vi "Update.vi"(8 "error in (no error)":errorcluster, 10 "Message in":refnum<class "UpdateMessage.lvclass">, 11 "DAQMH121119OrcaFlash in":refnum<class "DAQOrcaFlash.lvclass">) -> (0 "error out":errorcluster, 3 "DAQMH121119OrcaFlash out":refnum<class "DAQOrcaFlash.lvclass">)   [LabVIEW 2012, in "DAQOrcaFlash.lvclass"]
doc: "The update method processes the command 'update'. \n\nThe command 'update' is used for receiving new values to be set to the private data of the class. This could be seen as a public set method for setting new parameters to the private class data."
uses:
  DAQOrcaFlash.lvclass
  <vilib>/Distrio/Murmex/UpdateMessage/UpdateMessage.lvclass
  <vilib>/Distrio/Murmex/Murmex/Murmex.lvclass
  visualisation_line_cluster.ctl
  merit_factor_type.ctl
panel:
  # "This method is called when the UPDATE\ntrigger is sent. \n\nOverride this method when your component needs to\nrespond to this trigger. \n\nCall parent for proper implementation"
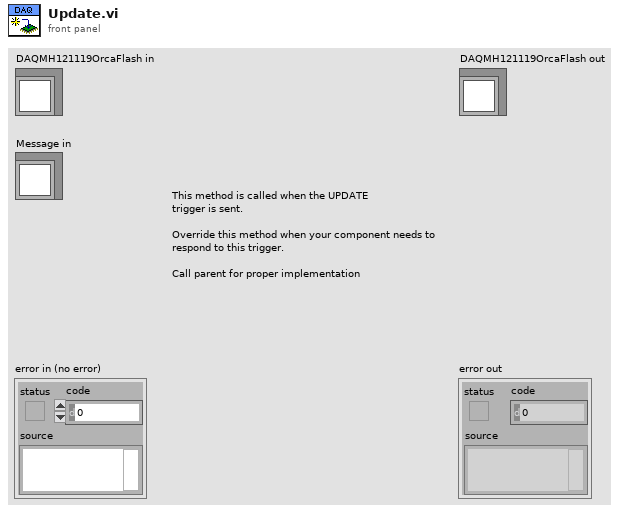
[diagram p1: front panel]
types:
  T1 = typedef "DAQOrcaFlash.lvclass/merit_factor_type.ctl" = enum16{"full frame intensity", "ROI beads", "Weber contrast", "Michelson contrast", "RMS contrast", "Line profile analysis", "ROI analysis", "FFT", "SNR", "5% brightest"}
  T2 = typedef "DAQOrcaFlash.lvclass/visualisation_line_cluster.ctl" = cluster{"direction":enum16{"horizontal", "vertical"}, "position":i32}
  T3 = typedef "IMAQ Image.ctl" = refnum<image>
  T4 = cluster{"Conversion Method":u32, "Minimum Value":i32, "Maximum Value":i32, "# Shifts":i32}
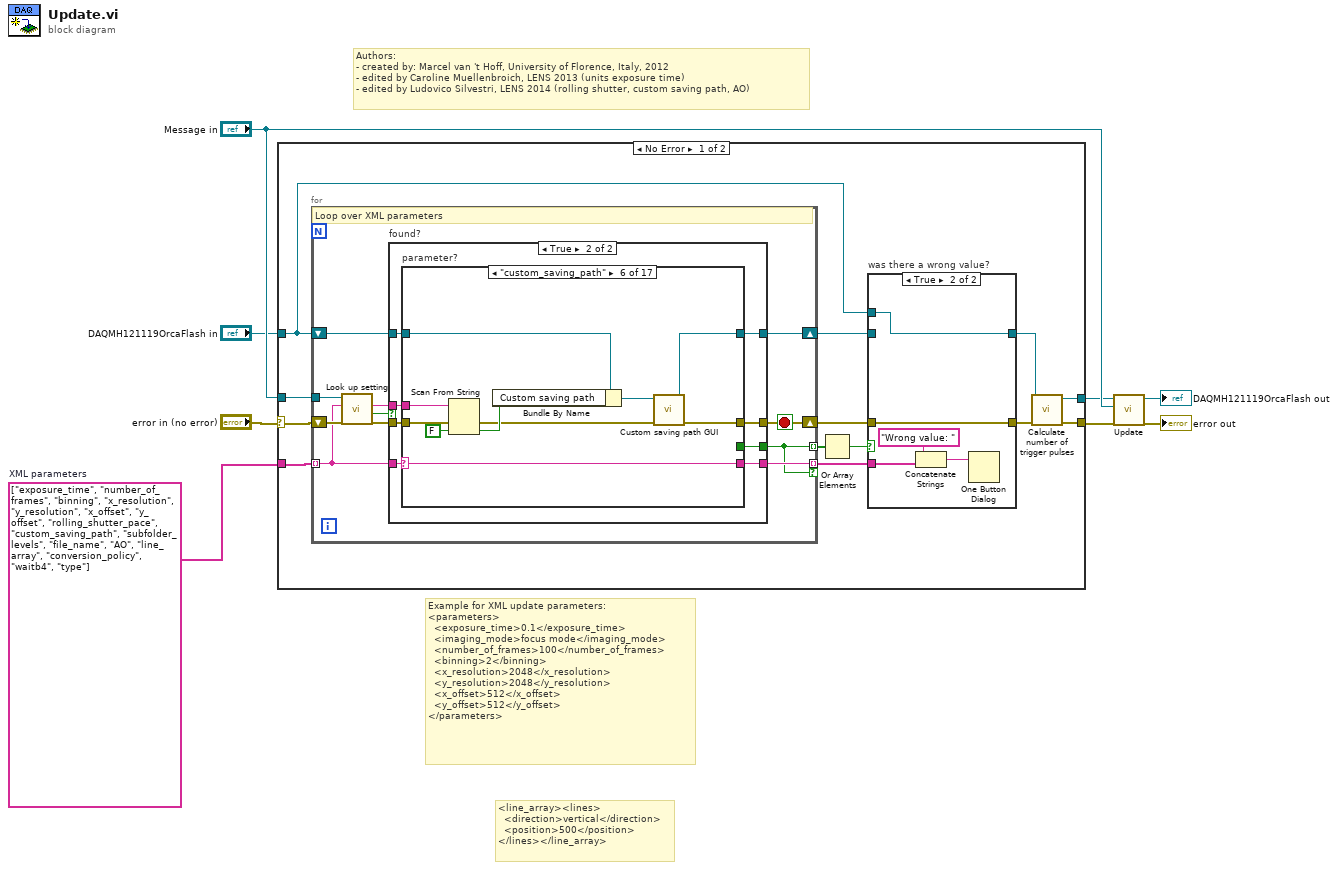
[diagram p0: block diagram]
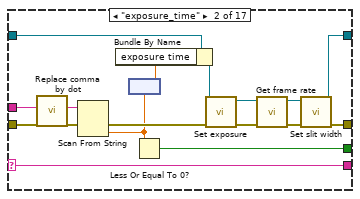
[diagram p5: hidden frame]
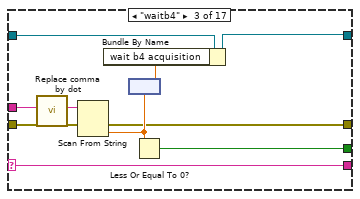
[diagram p6: hidden frame]
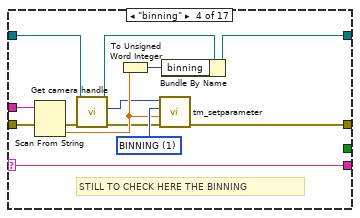
[diagram p7: hidden frame]
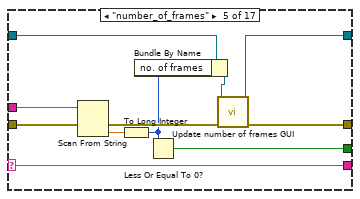
[diagram p8: hidden frame]
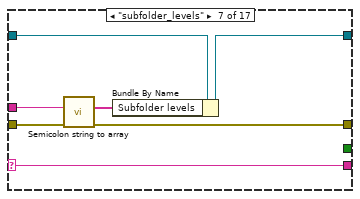
[diagram p9: hidden frame]
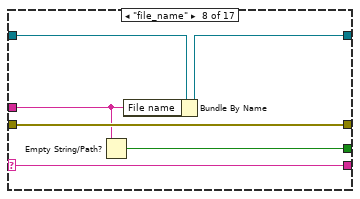
[diagram p10: hidden frame]
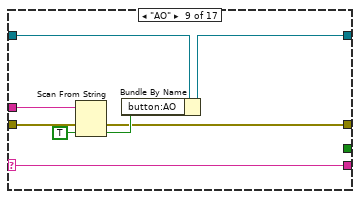
[diagram p11: hidden frame]
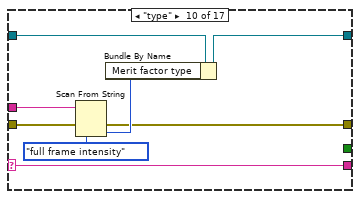
[diagram p12: hidden frame]
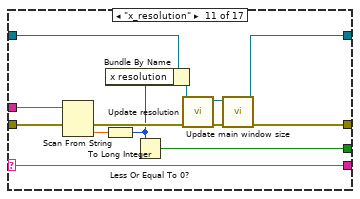
[diagram p13: hidden frame]
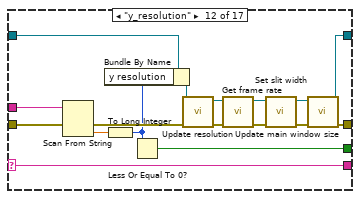
[diagram p14: hidden frame]
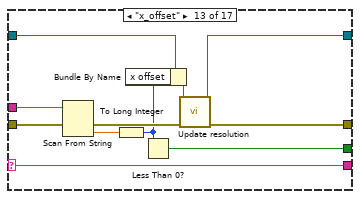
[diagram p15: hidden frame]
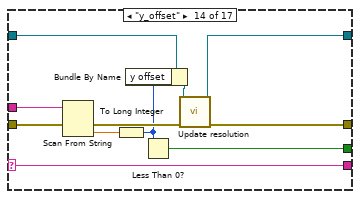
[diagram p16: hidden frame]
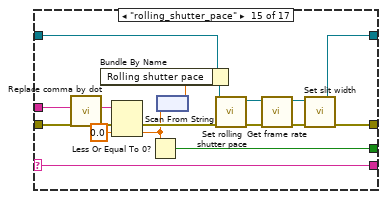
[diagram p17: hidden frame]
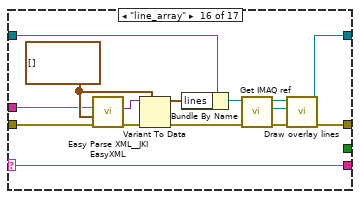
[diagram p18: hidden frame]
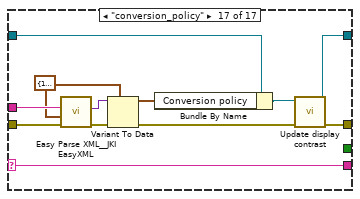
[diagram p19: hidden frame]
diagram:
  w8 = string[] ["exposure_time", "number_of_frames", "binning", "x_resolution", "y_resolution", "x_offset", "y_offset", "rolling_shutter_pace", "custom_saving_path", "subfolder_levels", "file_name", "AO", "line_array", "conversion_policy", "waitb4", "type"]  # XML parameters
  # "<line_array><lines>\n  <direction>vertical</direction>\n  <position>500</position>\n</lines></line_array>"
  # "Example for XML update parameters:\n<parameters>\n  <exposure_time>0.1</exposure_time>\n  <imaging_mode>focus mode</imaging_mode>\n  <number_of_frames>100</number_of_frames>\n  <binning>2</binning>\n  <x_resolution>2048</x_resolution>\n  <y_resolution>2048</y_resolution>\n  <x_offset>512</x_offset>\n  <y_offset>512</y_offset>\n</parameters>"
  # "Authors: \n- created by: Marcel van 't Hoff, University of Florence, Italy, 2012\n- edited by Caroline Muellenbroich, LENS 2013 (units exposure time)\n- edited by Ludovico Silvestri, LENS 2014 (rolling shutter, custom saving path, AO)"
  n1 = case shown="No Error" "error in (no error)" {
    selector: "error in (no error)" -> [w21 w240]
    tunnel: [w18 w240] -> w3
    tunnel: [w17 w239] -> w4
    tunnel: "DAQMH121119OrcaFlash in" -> [w14 w239]
    tunnel: "Message in" -> [w20 _]
    tunnel: w8 -> [w19 _]
    frame No Error {
      n2 = for "loop over parameters" {
        shift-right: [w37] -> w9
        shift-left: w21 -> [w35]
        shift-right: [w38] -> w12
        shift-left: w14 -> [w39]
        tunnel: w20 -> [w36]
        tunnel: w19 -> [w33] mode=indexing
        tunnel: [w29] -> w16 mode=indexing
        tunnel: [w30] -> w11 mode=indexing if=w29
        stop <- w37 stop-if-true
        # "Loop over XML parameters"
        n3 = call <vilib>:"Look up setting.vi"("error in (no error)"=w35, "tag name"=w33, "UpdateMessage in"=w36) -> ("error out"=w34:errorcluster, "found?"=w32:bool, "value"=w31:string)  [unwired: 5 in, 1 out]
        n4 = case "found?" shown="True" w32 {
          tunnel: w34 -> [w41 w50]
          tunnel: w31 -> [_ w49]
          tunnel: w33 -> [w40 w48]
          tunnel: w39 -> [w42 w47]
          tunnel: [w41 w46] -> w37
          tunnel: [w42 w45] -> w38
          tunnel: [_ w44] -> w29
          tunnel: [w40 w43] -> w30
          frame False {
          }
          frame True {
            # "XML parameter found?"
            n5 = case "parameter?" shown="\"custom_saving_path\"" w48 {
              selector: w48 -> [w51 w54 w72 w80 w95 w104 w114 w123 w127 w136 w143 w156 w173 w184 w195 w212 w227]
              tunnel: w50 -> [w52 w69 w79 w92 w102 w110 w118 w124 w133 w142 w153 w170 w181 w192 w210 w222 w235]
              tunnel: w49 -> [_ w68 w78 w91 w101 w111 w116 w122 w132 w141 w154 w171 w182 w193 w200 w223 w236]
              tunnel: w47 -> [w53 w59 w75 w84 w103 w113 w120 w126 w131 w140 w155 w172 w183 w194 w211 w221 w234]
              tunnel: [w52 w63 w71 w86 w98 w107 w117 w124 w128 w137 w149 w159 w177 w189 w205 w214 w231] -> w46
              tunnel: [w53 w62 w70 w90 w96 w105 w119 w125 w129 w138 w147 w161 w176 w187 w204 w216 w230] -> w45
              tunnel: [_ w55 w73 _ w93 _ _ w121 _ _ w144 w157 w174 w185 w196 _ _] -> w44
              tunnel: [w51 w54 w72 w80 w95 w104 w114 w123 w127 w136 w143 w156 w173 w184 w195 w212 w227] -> w43
              frame Default {
              }
              frame "exposure_time" {
                n6 = call <vilib>:"Replace comma by dot.vi"("input string"=w68) -> ("result string"=w66:string)  [unwired: 10 in]
                n7 = Scan From String(input string=w66, error in=w69) -> (error out=w57:errorcluster, output 1=w56:dbl)  [unwired: 3 in, 2 out]
                n8 = node(w56) -> (w67:dbl[unit])
                n9 = Bundle By Name(cluster=w59, "exposure time"=w67) -> (w58:refnum<class "DAQOrcaFlash.lvclass">)
                n10 = Less Or Equal To 0?(x=w56) -> (x <= 0?=w55:bool)
                n11 = call-dynamic "Set exposure.vi"("error in (no error)"=w57, "DAQOrcaFlash in"=w58) -> ("error out"=w61:errorcluster, "DAQOrcaFlash out"=w60:refnum<class "DAQOrcaFlash.lvclass">)  [unwired: 8 in]
                n12 = call-dynamic "Get frame rate.vi"("error in (no error)"=w61, "DAQOrcaFlash in"=w60) -> ("error out"=w64:errorcluster, "DAQOrcaFlash out"=w65:refnum<class "DAQOrcaFlash.lvclass">)  [unwired: 8 in]
                n13 = call-dynamic "Set slit width.vi"("error in (no error)"=w64, "DAQOrcaFlash in"=w65) -> ("error out"=w63:errorcluster, "DAQOrcaFlash out"=w62:refnum<class "DAQOrcaFlash.lvclass">)  [unwired: 8 in]
              }
              frame "waitb4" {
                n14 = call <vilib>:"Replace comma by dot.vi"("input string"=w78) -> ("result string"=w76:string)  [unwired: 10 in]
                n15 = Scan From String(input string=w76, error in=w79) -> (error out=w71:errorcluster, output 1=w74:dbl)  [unwired: 3 in, 2 out]
                n16 = node(w74) -> (w77:dbl[unit])
                n17 = Bundle By Name(cluster=w75, "wait b4 acquisition"=w77) -> (w70:refnum<class "DAQOrcaFlash.lvclass">)
                n18 = Less Or Equal To 0?(x=w74) -> (x <= 0?=w73:bool)
              }
              frame "binning" {
                w89 = 1 items=["BINNING"=1, "BITS PER CHANNEL"=2, "ACTIVE VIEW INDEX"=3, "CCD MODE"=4, "SENSOR MODE"=5, "READOUT MODE"=6, "EXPOSURE TIME"=7, "CONTRAST GAIN"=8, "CONTRAST OFFSET"=9, "LIGHT MODE"=10, "SENSITIVITY"=11, "WHITE BALANCE"=12, "PHOTON IMAGING MODE"=13, "HIGH DYNAMIC RANGE MODE"=14, "TRIGGER SOURCE"=15, "TRIGGER ACTIVE"=16, "TRIGGER MODE"=17, "TRIGGER POLARITY"=18, "TRIGGER GLOBAL EXPOSURE"=19, "FIRST TRIGGER BEHAVIOR"=20, "TRIGGER TIMES"=21, "OUTPUT TRIGGER POLARITY"=22, "OUTPUT TRIGGER DELAY"=23, "OUTPUT TRIGGER PERIOD"=24, "TEMPERATURE"=25, "TEMPERATURE TARGET"=26, "SENSOR COOLER FAN"=27, "MECHANICAL SHUTTER"=28, "BACK FOCUS POSITION"=29, "FRAMEBUNDLE MODE"=30, "FRAMEBUNDLE NUMBER"=31] ("Parameter")
                # "STILL TO CHECK HERE THE BINNING"
                n19 = Scan From String(input string=w91, error in=w92) -> (error out=w87:errorcluster, output 1=w88:dbl)  [unwired: 3 in, 2 out]
                n20 = call "Get camera handle.vi"("error in (no error)"=w87, "DAQMH121119OrcaFlash in"=w84) -> ("error out"=w85:errorcluster, "cam handle"=w82:u32, "DAQMH121119OrcaFlash out"=w83:refnum<class "DAQOrcaFlash.lvclass">)  [unwired: 7 in]
                n21 = To Unsigned Word Integer(number=w88) -> (unsigned 16bit integer=w81:u16)
                n22 = call <userlib>:"tm_setparameter.vi"("error in (no error)"=w85, "Value in"=w88, "Parameter"=w89, "Handle in"=w82) -> ("error out"=w86:errorcluster)  [unwired: 6 in, 1 out]
                n23 = Bundle By Name(cluster=w83, "binning"=w81) -> (w90:refnum<class "DAQOrcaFlash.lvclass">)
              }
              frame "number_of_frames" {
                n24 = Scan From String(input string=w101, error in=w102) -> (error out=w99:errorcluster, output 1=w100:dbl)  [unwired: 3 in, 2 out]
                n25 = To Long Integer(number=w100) -> (32bit integer=w94:i32)
                n26 = Bundle By Name(cluster=w103, "no. of frames"=w94) -> (w97:refnum<class "DAQOrcaFlash.lvclass">)
                n27 = Less Or Equal To 0?(x=w94) -> (x <= 0?=w93:bool)
                n28 = call-dynamic "Update number of frames GUI.vi"("error in (no error)"=w99, "DAQOrcaFlash in"=w97) -> ("error out"=w98:errorcluster, "DAQOrcaFlash out"=w96:refnum<class "DAQOrcaFlash.lvclass">)  [unwired: 8 in]
              }
              frame "custom_saving_path" {
                n29 = Scan From String(input string=w111, error in=w110, default 1=FALSE) -> (error out=w108:errorcluster, output 1=w109:bool)  [unwired: 2 in, 2 out]
                n30 = Bundle By Name(cluster=w113, "Custom saving path"=w109) -> (w106:refnum<class "DAQOrcaFlash.lvclass">)
                n31 = call-dynamic "Custom saving path GUI.vi"("error in (no error)"=w108, "DAQOrcaFlash in"=w106) -> ("error out"=w107:errorcluster, "DAQOrcaFlash out"=w105:refnum<class "DAQOrcaFlash.lvclass">)  [unwired: 8 in]
              }
              frame "subfolder_levels" {
                n32 = call "Semicolon string to array.vi"("error in"=w118, "Semicolon string"=w116) -> ("error out"=w117:errorcluster, "String array"=w115:string[])  [unwired: 8 in]
                n33 = Bundle By Name(cluster=w120, "Subfolder levels"=w115) -> (w119:refnum<class "DAQOrcaFlash.lvclass">)
              }
              frame "file_name" {
                n34 = Empty String/Path?(string/path=w122) -> (empty?=w121:bool)
                n35 = Bundle By Name(cluster=w126, "File name"=w122) -> (w125:refnum<class "DAQOrcaFlash.lvclass">)
              }
              frame "AO" {
                n36 = Scan From String(input string=w132, error in=w133, default 1=TRUE) -> (error out=w128:errorcluster, output 1=w130:bool)  [unwired: 2 in, 2 out]
                n37 = Bundle By Name(cluster=w131, "button:AO"=w130) -> (w129:refnum<class "DAQOrcaFlash.lvclass">)
              }
              frame "type" {
                n38 = Scan From String(input string=w141, error in=w142, default 1=merit_factor_type."full frame intensity" ("settings.Merit factor type")) -> (error out=w137:errorcluster, output 1=w139:T1)  [unwired: 2 in, 2 out]
                n39 = Bundle By Name(cluster=w140, "Merit factor type"=w139) -> (w138:refnum<class "DAQOrcaFlash.lvclass">)
              }
              frame "x_resolution" {
                n40 = Scan From String(input string=w154, error in=w153) -> (error out=w146:errorcluster, output 1=w152:dbl)  [unwired: 3 in, 2 out]
                n41 = To Long Integer(number=w152) -> (32bit integer=w145:i32)
                n42 = Bundle By Name(cluster=w155, "x resolution"=w145) -> (w151:refnum<class "DAQOrcaFlash.lvclass">)
                n43 = Less Or Equal To 0?(x=w145) -> (x <= 0?=w144:bool)
                n44 = call "Update resolution.vi"("error in (no error)"=w146, "DAQMH121119OrcaFlash in"=w151) -> ("error out"=w150:errorcluster, "DAQMH121119OrcaFlash out"=w148:refnum<class "DAQOrcaFlash.lvclass">)  [unwired: 8 in]
                n45 = call "Update main window size.vi"("error in (no error)"=w150, "DAQOrcaFlash in"=w148) -> ("error out"=w149:errorcluster, "DAQOrcaFlash out"=w147:refnum<class "DAQOrcaFlash.lvclass">)  [unwired: 8 in]
              }
              frame "y_resolution" {
                n46 = Scan From String(input string=w171, error in=w170) -> (error out=w168:errorcluster, output 1=w169:dbl)  [unwired: 3 in, 2 out]
                n47 = To Long Integer(number=w169) -> (32bit integer=w158:i32)
                n48 = Bundle By Name(cluster=w172, "y resolution"=w158) -> (w167:refnum<class "DAQOrcaFlash.lvclass">)
                n49 = Less Or Equal To 0?(x=w158) -> (x <= 0?=w157:bool)
                n50 = call "Update resolution.vi"("error in (no error)"=w168, "DAQMH121119OrcaFlash in"=w167) -> ("error out"=w164:errorcluster, "DAQMH121119OrcaFlash out"=w163:refnum<class "DAQOrcaFlash.lvclass">)  [unwired: 8 in]
                n51 = call-dynamic "Get frame rate.vi"("error in (no error)"=w164, "DAQOrcaFlash in"=w163) -> ("error out"=w166:errorcluster, "DAQOrcaFlash out"=w165:refnum<class "DAQOrcaFlash.lvclass">)  [unwired: 8 in]
                n52 = call-dynamic "Set slit width.vi"("error in (no error)"=w166, "DAQOrcaFlash in"=w165) -> ("error out"=w160:errorcluster, "DAQOrcaFlash out"=w162:refnum<class "DAQOrcaFlash.lvclass">)  [unwired: 8 in]
                n53 = call "Update main window size.vi"("error in (no error)"=w160, "DAQOrcaFlash in"=w162) -> ("error out"=w159:errorcluster, "DAQOrcaFlash out"=w161:refnum<class "DAQOrcaFlash.lvclass">)  [unwired: 8 in]
              }
              frame "x_offset" {
                n54 = Scan From String(input string=w182, error in=w181) -> (error out=w179:errorcluster, output 1=w180:dbl)  [unwired: 3 in, 2 out]
                n55 = To Long Integer(number=w180) -> (32bit integer=w175:i32)
                n56 = Bundle By Name(cluster=w183, "x offset"=w175) -> (w178:refnum<class "DAQOrcaFlash.lvclass">)
                n57 = Less Than 0?(x=w175) -> (x < 0?=w174:bool)
                n58 = call "Update resolution.vi"("error in (no error)"=w179, "DAQMH121119OrcaFlash in"=w178) -> ("error out"=w177:errorcluster, "DAQMH121119OrcaFlash out"=w176:refnum<class "DAQOrcaFlash.lvclass">)  [unwired: 8 in]
              }
              frame "y_offset" {
                n59 = Scan From String(input string=w193, error in=w192) -> (error out=w190:errorcluster, output 1=w191:dbl)  [unwired: 3 in, 2 out]
                n60 = To Long Integer(number=w191) -> (32bit integer=w186:i32)
                n61 = Bundle By Name(cluster=w194, "y offset"=w186) -> (w188:refnum<class "DAQOrcaFlash.lvclass">)
                n62 = Less Than 0?(x=w186) -> (x < 0?=w185:bool)
                n63 = call "Update resolution.vi"("error in (no error)"=w190, "DAQMH121119OrcaFlash in"=w188) -> ("error out"=w189:errorcluster, "DAQMH121119OrcaFlash out"=w187:refnum<class "DAQOrcaFlash.lvclass">)  [unwired: 8 in]
              }
              frame "rolling_shutter_pace" {
                n64 = call <vilib>:"Replace comma by dot.vi"("input string"=w200) -> ("result string"=w199:string)  [unwired: 10 in]
                n65 = Scan From String(input string=w199, error in=w210, default 1=sgl 0.0 ("default value 1")) -> (error out=w209:errorcluster, output 1=w197:sgl)  [unwired: 2 in, 2 out]
                n66 = Less Or Equal To 0?(x=w197) -> (x <= 0?=w196:bool)
                n67 = node(w197) -> (w198:sgl[unit])
                n68 = Bundle By Name(cluster=w211, "Rolling shutter pace"=w198) -> (w208:refnum<class "DAQOrcaFlash.lvclass">)
                n69 = call-dynamic "Set rolling shutter pace.vi"("error in (no error)"=w209, "DAQOrcaFlash in"=w208) -> ("error out"=w207:errorcluster, "DAQOrcaFlash out"=w203:refnum<class "DAQOrcaFlash.lvclass">)  [unwired: 8 in]
                n70 = call-dynamic "Get frame rate.vi"("error in (no error)"=w207, "DAQOrcaFlash in"=w203) -> ("error out"=w206:errorcluster, "DAQOrcaFlash out"=w202:refnum<class "DAQOrcaFlash.lvclass">)  [unwired: 8 in]
                n71 = call-dynamic "Set slit width.vi"("error in (no error)"=w206, "DAQOrcaFlash in"=w202) -> ("error out"=w205:errorcluster, "DAQOrcaFlash out"=w204:refnum<class "DAQOrcaFlash.lvclass">)  [unwired: 8 in]
              }
              frame "line_array" {
                w225 = T2[] [] ("lines")
                n72 = call <vilib>:"Easy Parse XML__JKI EasyXML.vi"("error in (no error)"=w222, "LabVIEW Data (Type)"=w225, "XML String"=w223) -> ("error out"=w226:errorcluster, "LabVIEW Data"=w224:variant)  [unwired: 7 in]
                n73 = Variant To Data(error in=w226, type=w225, Variant=w224) -> (data=w220:T2[], error out=w219:errorcluster)
                n74 = Bundle By Name(cluster=w221, "lines"=w220) -> (w217:refnum<class "DAQOrcaFlash.lvclass">)
                n75 = call "Get IMAQ ref.vi"("error in (no error)"=w219, "DAQMH121119OrcaFlash in"=w217) -> ("error out"=w215:errorcluster, "IMAQ reference"=w213:T3, "DAQMH121119OrcaFlash out"=w218:refnum<class "DAQOrcaFlash.lvclass">)  [unwired: 7 in]
                n76 = call "Draw overlay lines.vi"("error in (no error)"=w215, "IMAQ reference"=w213, "DAQOrcaFlash in"=w218) -> ("error out"=w214:errorcluster, "DAQOrcaFlash out"=w216:refnum<class "DAQOrcaFlash.lvclass">)  [unwired: 6 in, 1 out]
              }
              frame "conversion_policy" {
                w228 = T4 {"Conversion Method"=10, "Minimum Value"=0, "Maximum Value"=1000, "# Shifts"=0} ("Conversion policy")
                n77 = call <vilib>:"Easy Parse XML__JKI EasyXML.vi"("error in (no error)"=w235, "LabVIEW Data (Type)"=w228, "XML String"=w236) -> ("error out"=w238:errorcluster, "LabVIEW Data"=w237:variant)  [unwired: 7 in]
                n78 = Variant To Data(error in=w238, type=w228, Variant=w237) -> (data=w233:T4, error out=w232:errorcluster)
                n79 = Bundle By Name(cluster=w234, "Conversion policy"=w233) -> (w229:refnum<class "DAQOrcaFlash.lvclass">)
                n80 = call-dynamic "Update display contrast.vi"("error in (no error)"=w232, "DAQOrcaFlash in"=w229) -> ("error out"=w231:errorcluster, "DAQOrcaFlash out"=w230:refnum<class "DAQOrcaFlash.lvclass">)  [unwired: 8 in]
              }
            }
          }
        }
      }
      n81 = Or Array Elements(Boolean array=w16) -> (logical OR=w15:bool)
      n82 = case "was there a wrong value?" shown="True" w15 {
        tunnel: w14 -> [_ w28]
        tunnel: [w23 w28] -> w13
        tunnel: w12 -> [w23 _]
        tunnel: w11 -> [_ w27]
        tunnel: [w22 w24] -> w10
        tunnel: w9 -> [w22 w24]
        frame False {
        }
        frame True {
          n83 = Concatenate Strings("Wrong value: " ("message"), w27) -> (w25:string)
          n84 = One Button Dialog(message=w25) -> ()  [unwired: 1 in, 1 out]
        }
      }
      n85 = call "Calculate number of trigger pulses.vi"("error in (no error)"=w10, "DAQOrcaFlash in"=w13) -> ("error out"=w18:errorcluster, "DAQOrcaFlash out"=w17:refnum<class "DAQOrcaFlash.lvclass">)  [unwired: 8 in]
    }
    frame Error {
    }
  }
  n86 = call-parent "Update.vi"("error in (no error)"=w3, "Message in"="Message in", "Murmex in"=w4) -> ("error out"=→"error out":errorcluster, "Murmex out"=→"DAQMH121119OrcaFlash out":refnum<class "DAQOrcaFlash.lvclass">)  [unwired: 7 in]
